vi "extract-hiearchy-from-path.vi"(10 "base":path, 11 "location":path) -> (3 "Array":string[](array[string]), 5 "relative path":path)   [LabVIEW 2014]
panel:
  out "vi path out":path
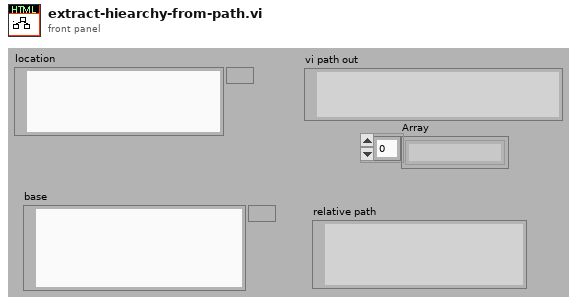
[diagram p1: front panel]
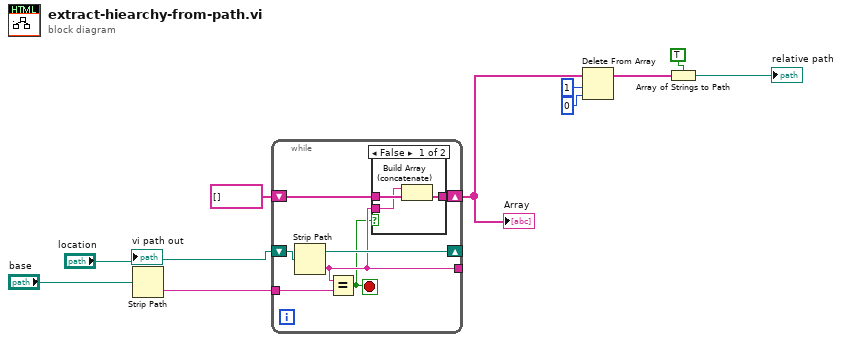
[diagram p0: block diagram]
diagram:
  n1 = Strip Path(path="base") -> (name=w7:string)  [unwired: 1 out]
  n2 = while {
    shift-right: [w16] -> _
    shift-left: "location" -> [w17]
    tunnel: w7 -> [w15]
    tunnel: [w14] -> _
    shift-right: [w13] -> w5
    shift-left: string[] [] -> [w12]
    stop <- w11 stop-if-true
    n3 = Strip Path(path=w17) -> (stripped path=w16:path, name=w14:string)
    n4 = Equal?(x=w14, y=w15) -> (x = y?=w11:bool)
    n5 = case shown="False" w11 {
      tunnel: w14 -> [w18 _]
      tunnel: [w20 w21] -> w13
      tunnel: w12 -> [w19 w21]
      frame False {
        n6 = Build Array (concatenate)(w18, w19) -> (w20:string[])
      }
      frame True {
      }
    }
  }
  "Array" <- w5
  n7 = Delete From Array(array=w5, length=1, index=0) -> (array with subset deleted=w2:string[])  [unwired: 1 out]
  n8 = Array of Strings to Path(0:w2, 1:TRUE ("relative")) -> (2:→"relative path":path)
  "vi path out" <- "location"
